vi "HillCipherEncryption.vi"(6 "Encryption Key":u8[][](array[numeric])=[[25, 2, 21], [4, 12, 6], [8, 41, 32]], 10 "Operation":enum16{"Encrypt", "Decrypt", "Decrypt from Hex"}(ring), 11 "Input String":string) -> (1 "Invalid encryption key":bool, 2 "Output String (Hex)":string, 3 "Output String":string)   [LabVIEW 2020]
uses:
  <vilib>/Analysis/Matrix/Datatypes/RealMatrix.ctl
  <vilib>/Analysis/baseanly.llb/Real A x B.vi
  <vilib>/Analysis/baseanly.llb/A x Vector.vi
  <vilib>/Analysis/baseanly.llb/Real Inverse Matrix.vi
  <vilib>/Analysis/Matrix/Comparison/Not Equal/Not Equal - RM,RM.vi
  <vilib>/Analysis/NI_AALBase.lvlib
  <vilib>/Analysis/Matrix/NI_Matrix.lvlib
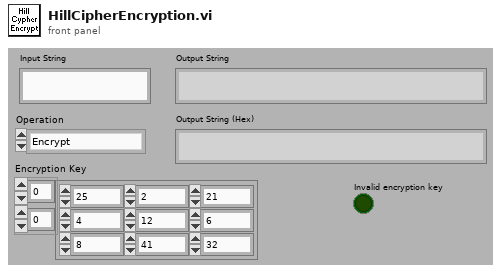
[diagram p1: front panel]
types:
  T1 = typedef "NI_Matrix.lvlib/RealMatrix.ctl" = dbl[][]
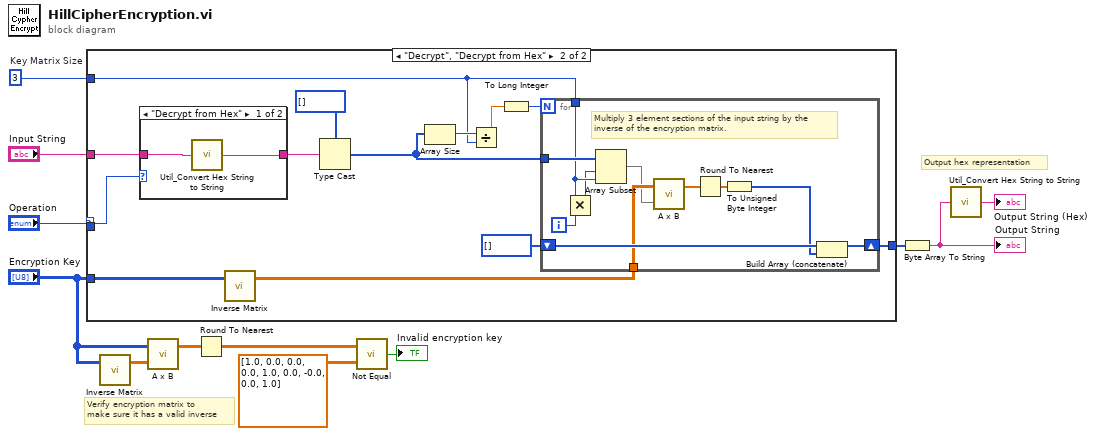
[diagram p0: block diagram]
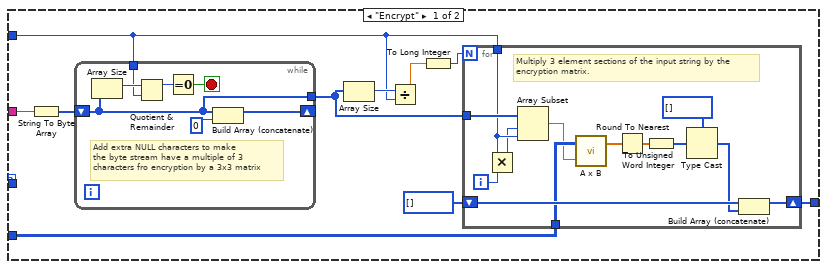
[diagram p2: hidden frame]
diagram:
  w11 = 3  # Key Matrix Size
  # "Output hex representation"
  # "Verify encryption matrix to\nmake sure it has a valid inverse"
  n1 = case shown="\"Decrypt\", \"Decrypt from Hex\"" "Operation" {
    selector: "Operation" -> [w14 w46]
    tunnel: "Input String" -> [w23 w45]
    tunnel: [w15 w51] -> w4
    tunnel: "Encryption Key" -> [w13 w50]
    tunnel: [w14 w46] -> _
    tunnel: w11 -> [w17 w52]
    frame "Encrypt" {
      n2 = String To Byte Array(string=w23) -> (unsigned byte array=w18:u8[])
      n3 = while {
        shift-right: [w30] -> _
        shift-left: w18 -> [w24]
        tunnel: w17 -> [w27]
        tunnel: [w24] -> w16
        stop <- w25 stop-if-true
        # "Add extra NULL characters to make\nthe byte stream have a multiple of 3\ncharacters fro encryption by a 3x3 matrix"
        n4 = Array Size(array=w24) -> (size(s)=w28:i32)
        n5 = Quotient & Remainder(x=w28, y=w27) -> (x-y*floor(x/y)=w26:i32)  [unwired: 1 out]
        n6 = Equal To 0?(x=w26) -> (x = 0?=w25:bool)
        n7 = Build Array (concatenate)(w24, u8 0) -> (w30:u8[])
      }
      n8 = Array Size(array=w16) -> (size(s)=w22:i32)
      n9 = Divide(x=w22, y=w17) -> (x/y=w21:dbl)
      n10 = To Long Integer(number=w21) -> (32bit integer=w20:i32)
      n11 = for {
        N: w20 -> [_]
        tunnel: w16 -> [w42]
        tunnel: w17 -> [w39]
        shift-right: [w41] -> w15
        shift-left: u8[] [] -> [w40]
        tunnel: w13 -> [w37]
        i -> [w43]
        # "Multiply 3 element sections of the input string by the\nencryption matrix."
        n12 = Multiply(x=w39, y=w43) -> (x*y=w38:i32)
        n13 = Array Subset(array=w42, index=w38, length=w39) -> (w36:u8[])
        n14 = call-poly <vilib>:"A x B.vi"("Vector"=w36, "A"=w37) -> ("A x Vector"=w35:dbl[])  [unwired: 1 out]
        n15 = Round To Nearest(number=w35) -> (nearest integer value=w34:dbl[])
        n16 = To Unsigned Word Integer(number=w34) -> (unsigned 16bit integer=w33:u16[])
        n17 = Type Cast(type=u8[] [], x=w33) -> (*(type *) &x=w31:u8[])
        n18 = Build Array (concatenate)(w40, w31) -> (w41:u8[])
      }
    }
    frame "Decrypt", "Decrypt from Hex" {
      n19 = case shown="\"Decrypt from Hex\"" w46 {
        tunnel: [w57 w59] -> w44
        tunnel: w45 -> [w58 w59]
        frame "Decrypt from Hex" {
          n20 = call "Util_Convert Hex String to String.vi"("Hex String"=w58) -> ("String"=w57:string)  [unwired: 4 in]
        }
        frame "Decrypt", Default {
        }
      }
      n21 = call-poly <vilib>:"Inverse Matrix.vi"("Input Matrix"=w50) -> ("Inverse Matrix"=w49:T1)  [unwired: 1 in, 1 out]
      n22 = Type Cast(type=u16[] [], x=w44) -> (*(type *) &x=w47:u16[])
      n23 = Array Size(array=w47) -> (size(s)=w56:i32)
      n24 = Divide(x=w56, y=w52) -> (x/y=w55:dbl)
      n25 = To Long Integer(number=w55) -> (32bit integer=w54:i32)
      n26 = for {
        N: w54 -> [_]
        tunnel: w47 -> [w69]
        tunnel: w52 -> [w66]
        shift-right: [w68] -> w51
        shift-left: u8[] [] -> [w67]
        tunnel: w49 -> [w64]
        i -> [w70]
        # "Multiply 3 element sections of the input string by the\ninverse of the encryption matrix."
        n27 = Multiply(x=w66, y=w70) -> (x*y=w65:i32)
        n28 = Array Subset(array=w69, index=w65, length=w66) -> (w63:u16[])
        n29 = call-poly <vilib>:"A x B.vi"("Vector"=w63, "A"=w64) -> ("A x Vector"=w62:dbl[])  [unwired: 1 out]
        n30 = Round To Nearest(number=w62) -> (nearest integer value=w61:dbl[])
        n31 = To Unsigned Byte Integer(number=w61) -> (unsigned 8bit integer=w60:u8[])
        n32 = Build Array (concatenate)(w67, w60) -> (w68:u8[])
      }
    }
  }
  n33 = call-poly <vilib>:"Inverse Matrix.vi"("Input Matrix"="Encryption Key") -> ("Inverse Matrix"=w9:T1)  [unwired: 1 in, 1 out]
  n34 = call-poly <vilib>:"A x B.vi"("B"=w9, "A"="Encryption Key") -> ("A x B"=w8:T1)  [unwired: 1 out]
  n35 = Round To Nearest(number=w8) -> (nearest integer value=w7:T1)
  n36 = call-poly <vilib>:"Not Equal.vi"("Real Matrix B"=T1 [[1.0, 0.0, 0.0], [0.0, 1.0, 0.0], [-0.0, 0.0, 1.0]] ("nearest integer value"), "Real Matrix A"=w7) -> ("A != B?"=→"Invalid encryption key":bool)
  n37 = Byte Array To String(unsigned byte array=w4) -> (string=w1:string)
  "Output String" <- w1
  n38 = call "Util_Convert Hex String to String.vi"("Hex String"=w1) -> ("String"=→"Output String (Hex)":string)  [unwired: 4 in]
